vi "Preferences.vi"() -> ()   [LabVIEW 2012]
panel:
  in  "Restore Defaults":bool
  in  "Cancel":bool
  in  "OK":bool
  in  "Tab Control":enum32{"General", "Apatite FT", "(U-Th)/He"}(tab)
  in  "DefaultMaxTime":dbl caption="Time-temperature history default maximum time (Ma):"
  in  "DefaultMaxTemp":dbl caption="Time-temperature history default maximum temperature (°C):"
  in  "KparAxisMax":dbl caption=":"
  in  "AxisKpar":string(combo) caption="Defaul axis maximum for plotting kinetic parameter:"
  in  "DparConvInt":dbl caption="µm"
  in  "DparConvSlope":dbl caption="Carlson et al. (1999) (µm) ="
  in  "LocInt":dbl
  out "LocKpar":string
  in  "LocSlope":dbl caption="Lo (c) ="
  out "EtchMethod":string caption="Etch method:"
  in  "LomInt":dbl
  in  "LoKpar":string(combo)
  in  "LomSlope":dbl caption="Lo (mean):"
  in  "DefConstLo":dbl caption="Default constant value (µm):"
  in  "DefaultLoSource":string(combo) caption="Default initial track length source:"
  in  "DefCfIrrad":string(combo) caption="Default Cf-irrad. usage:"
  in  "DefZetaMode":string(combo) caption="Default zeta mode:"
  in  "DefLengthGOF":string(combo) caption="Default length GOF:"
  in  "DefStdLenRed":dbl caption="Default length reduction in standard:"
  in  "DefAgeReporting":string(combo) caption="Default age uncertainty reporting:"
  in  "DefDoCAxisProj":string(combo) caption="Default c-axis projection usage:"
  in  "KparValue":dbl caption="Value:"
  in  "DefKpar":string(combo) caption="Default kinetic parameter:"
  in  "DefCAxisProjModel":string(combo) caption="Default c-axis projection model:"
  in  "DefaultAnnealingModel":string(combo) caption="Default annealing model:"
  in  "DefaultOtherDinf":dbl caption="cm²/sec"
  in  "DefaultOtherDinfType":string(combo)
  in  "DefaultOtherActivationEnergy":dbl caption="Activation Energy (E):"
  in  "DefaultOtherMineral":string(combo) caption="Mineral:"
  in  "DefaultGeometry":string(combo) caption="Geometry:"
  in  "DefaultAlphaCorr":string(combo) caption="Default alpha correction:"
  in  "DefaultRadius":dbl caption="Default radius:"
  in  "DefaultAlpha":string(combo) caption="Default alpha calculation:"
  in  "DefaultAgeToReport":string(combo) caption="Default age to report:"
  in  "DefaultDiffCalib":string(combo) caption="Default diffusion calibration:"
  # "Defaults for new models:"
  # "(also defines Lo etch method)"
  # "Initial track length estimation:"
  # "*"
  # "+"
  # "+"
  # "*"
  # "Kinetic parameter information:"
  # "* My Dpar +"
  # "Dpar conversion:"
  # "µm"
  # "Default \"Other\" calibration parameters"
  # "kcal/mol"
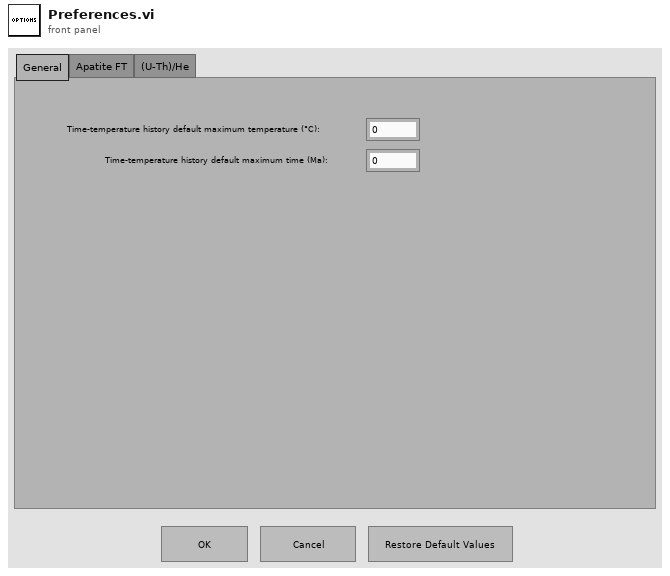
[diagram p1: front panel]
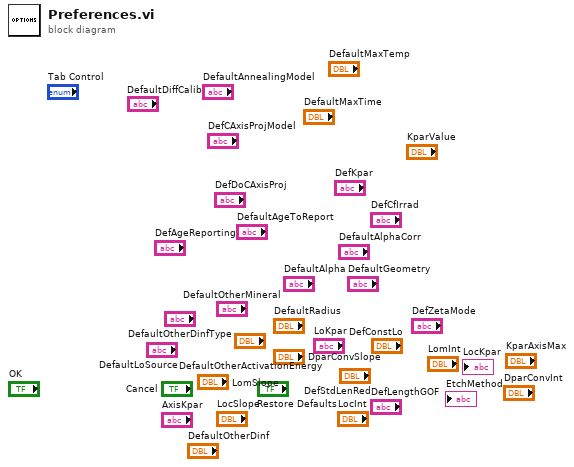
[diagram p0: block diagram]
diagram:
